vi "AlliGator Load HDF5 FLI Dataset Information.vi"(8 "Error In":errorcluster, 11 "File Path":path) -> (0 "error out":errorcluster, 1 "Data Description":string, 2 "Metadata":string, 3 "FLI Data File Information":T1, 4 "elapsed (relative) seconds":dbl)   [LabVIEW 2021, in "AlliGator HDF5.lvlib"]
doc: "Loads HDF5 FLI dataset information."
uses:
  AlliGator HDF5.lvlib
  AlliGator FLI Data File Information.ctl
  Phasor/Phasor Fluorescence Lifetime Parameters v3.ctl
  Files/AlliGator FLI Dataset Type.ctl
  AlliGator HDF5 FLI File Loading Information v0.6.ctl
  AlliGator HDF5 FLI File Loading Information v0.2.ctl
  Phasor/Fluorescence Lifetime Parameters.ctl
  SwissSPAD/SwissSPAD Live_Image ROI Information.ctl
  Source Image/AlliGator Image Binning Options.ctl
  Phasor/Phasor Fluorescence Lifetime Parameters v2.ctl
  <vilib>/addons/h5labview2/base/lib_path.vi
  <vilib>/addons/h5labview2/base/H5Equery.vi
  <vilib>/Utility/error.llb/Error Cluster From Error Code.vi
  AlliGator Load Single HDF5 Gate Image v 0.2b.vi
  AlliGator Load Single HDF5 Gate Image v 0.3b.vi
  AlliGator Load Single Gate Image from HDF5 v 0.6b.vi
  <vilib>/addons/h5labview2/base/hid_t.ctl
  <vilib>/addons/h5labview2/dataset/H5Dread.llb/H5Dread.xnode
  <vilib>/ErrorRing/Error Ring.xnode
  <vilib>/addons/h5labview2/file/H5F.lvlib
  <vilib>/addons/h5labview2/group/H5G.lvlib
  Time/Time.lvlib
  Phasor/Phasor.lvlib
  SwissSPAD/SwissSPAD Live.lvlib
  Source Image/AlliGator Source Image.lvlib
  Files/AlliGator Files.lvlib
  Variant/Variant.lvlib
panel:
  # "see the AlliGator License on the block diagram (Ctrl+E or Window:Show Block Diagram)"
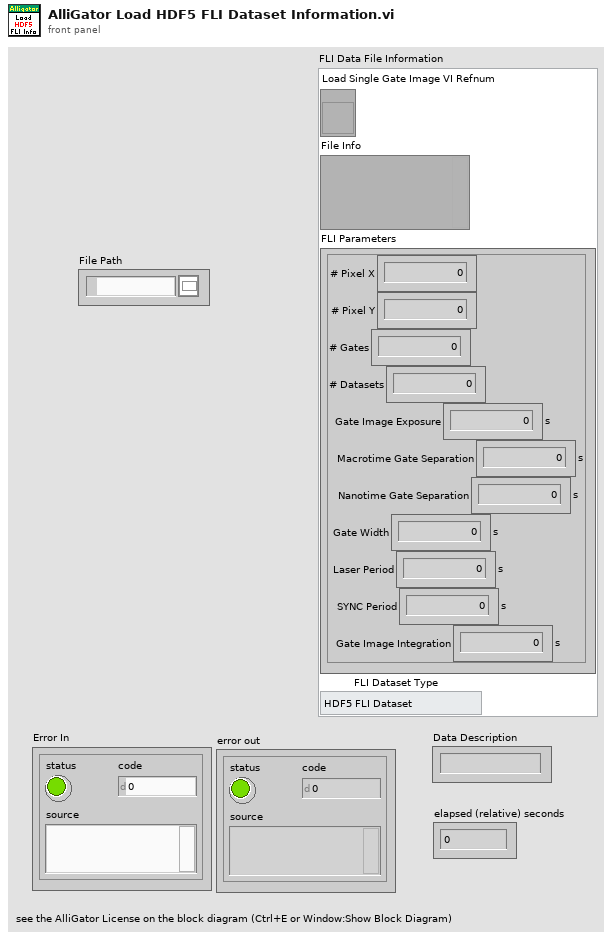
[diagram p1: front panel]
types:
  T1 = typedef "AlliGator HDF5.lvlib/AlliGator FLI Data File Information.ctl" = cluster{"Load Single Gate Image VI Refnum":refnum<vi>, "File Info":variant, "FLI Parameters":T2, "FLI Dataset Type":T3}
  T2 = typedef "Phasor.lvlib/Phasor Fluorescence Lifetime Parameters v3.ctl" = cluster{"# Pixel X":i32, "# Pixel Y":i32, "# Gates":i32, "# Datasets":i32, "Gate Image Exposure":dbl[unit], "Macrotime Gate Separation":dbl[unit], "Nanotime Gate Separation":dbl[unit], "Gate Width":dbl[unit], "Laser Period":dbl[unit], "SYNC Period":dbl[unit], "Gate Image Integration":dbl[unit]}
  T3 = typedef "AlliGator Files.lvlib/AlliGator FLI Dataset Type.ctl" = enum16{"HDF5 FLI Dataset", "Gate Image Folder", ".sdt FLI Dataset (Becker & Hickl)", ".ptu FLI Dataset (PicoQuant)", "SS1 FLI Dataset", "SS2 FLI Dataset", "I/m/phi Dataset", ".bin FLI Dataset (PicoQuant Binned)", ".bin FLI Dataset (Piccolo Binned)"}
  T4 = typedef "AlliGator HDF5.lvlib/AlliGator HDF5 FLI File Loading Information v0.6.ctl" = cluster{"HDF5 File Path":path, "Data Type":string, "# Datasets in Series":i32, "Dataset ID in Series":i32, "Channel Names":string[]}
  T5 = typedef "Phasor.lvlib/Fluorescence Lifetime Parameters.ctl" = cluster{"# Pixel X":i32, "# Pixel Y":i32, "# Gates":i32, "# Datasets":i32, "Exposure/Gate":dbl[unit], "Macrotime Gate Separation":dbl[unit], "Nanotime Gate Separation":dbl[unit], "Gate Duration":dbl[unit], "Laser Period":dbl[unit]}
  T6 = typedef "AlliGator HDF5.lvlib/AlliGator HDF5 FLI File Loading Information v0.2.ctl" = cluster{"HDF5 File Path":path}
  T7 = typedef "AlliGator Source Image.lvlib/AlliGator Image Binning Options.ctl" = cluster{"Use Image Binning":bool, "X Bin":i32, "Y Bin":i32}
  T8 = typedef "SwissSPAD Live.lvlib/SwissSPAD Live_Image ROI Information.ctl" = cluster{"Save ROI Only":bool, "Left":u16, "Top":u16, "Right":u16, "Bottom":u16, "Use Current ROI":bool}
  T9 = typedef "Phasor.lvlib/Phasor Fluorescence Lifetime Parameters v2.ctl" = cluster{"# Pixel X":i32, "# Pixel Y":i32, "# Gates":i32, "# Datasets":i32, "Exposure/Gate":dbl[unit], "Macrotime Gate Separation":dbl[unit], "Nanotime Gate Separation":dbl[unit], "Gate Duration":dbl[unit], "Laser Period":dbl[unit], "SYNC Period":dbl[unit]}
  T10 = typedef "hid_t.ctl" = i64
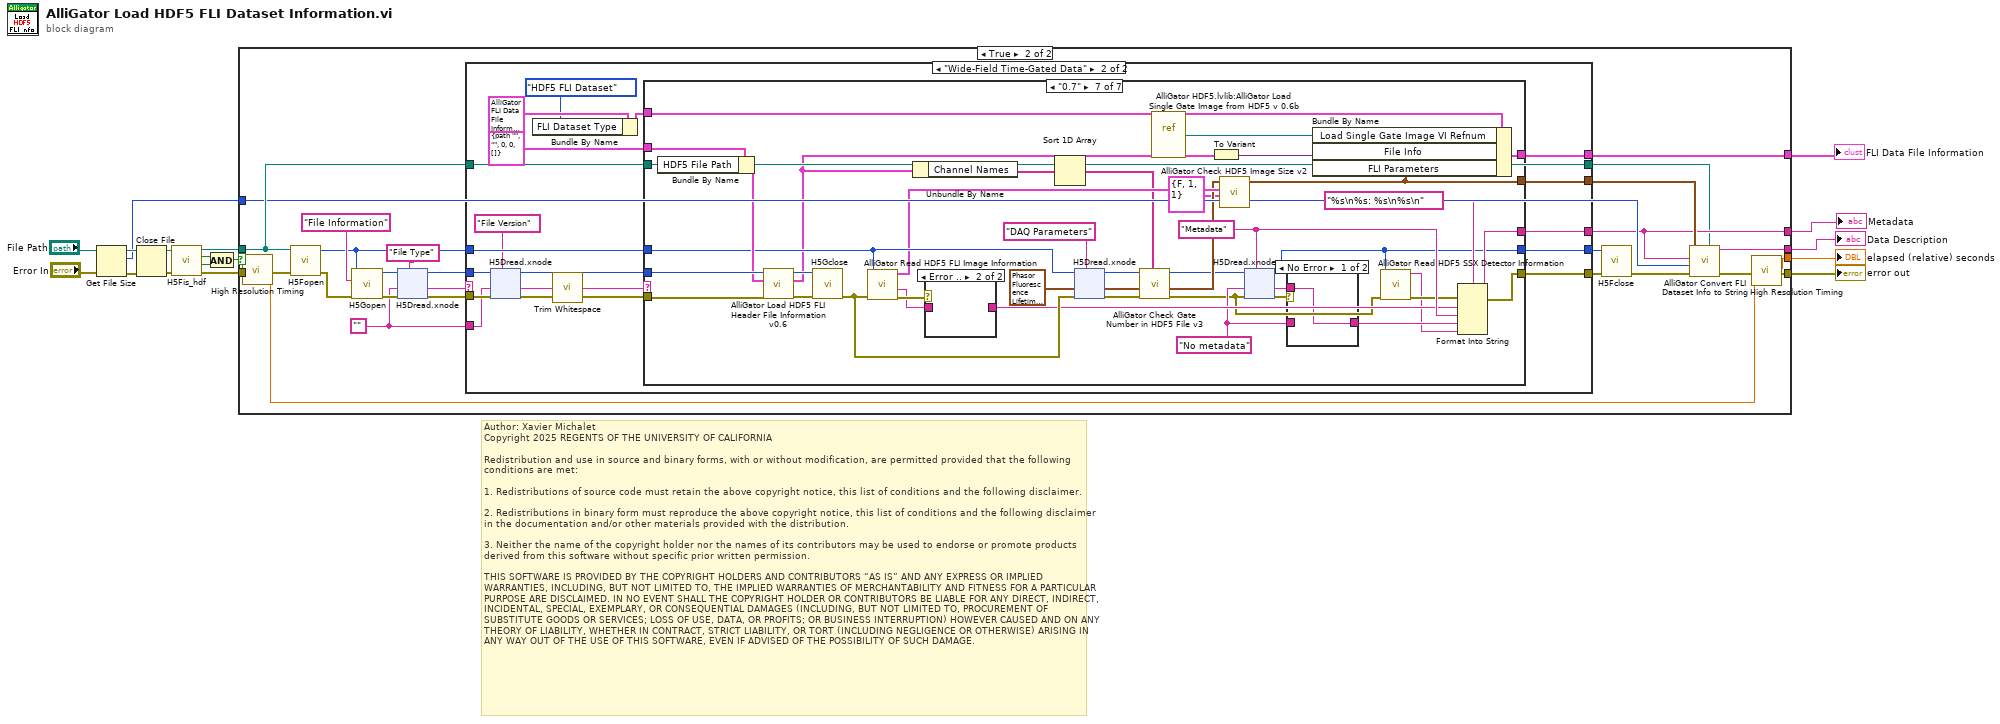
[diagram p0: block diagram]
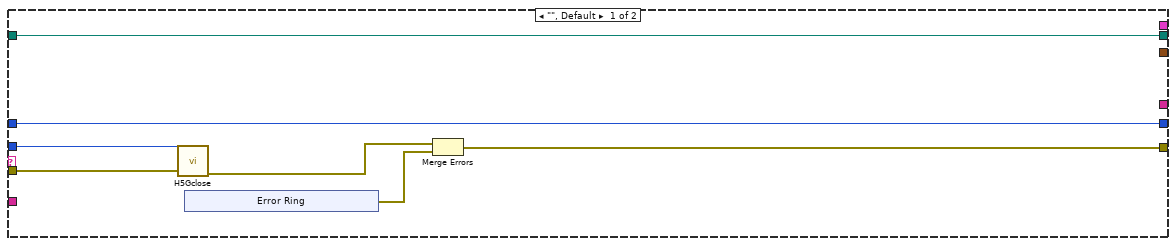
[diagram p3: hidden frame]
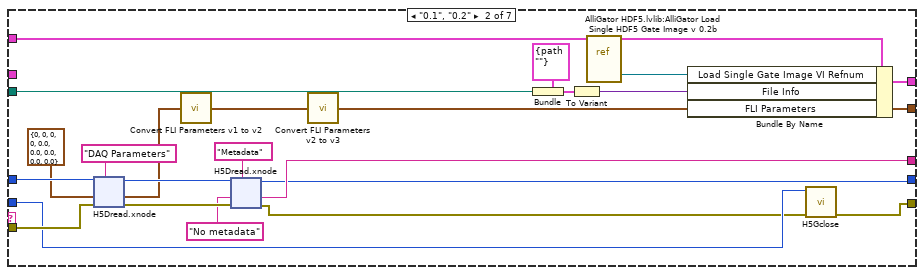
[diagram p5: hidden frame]
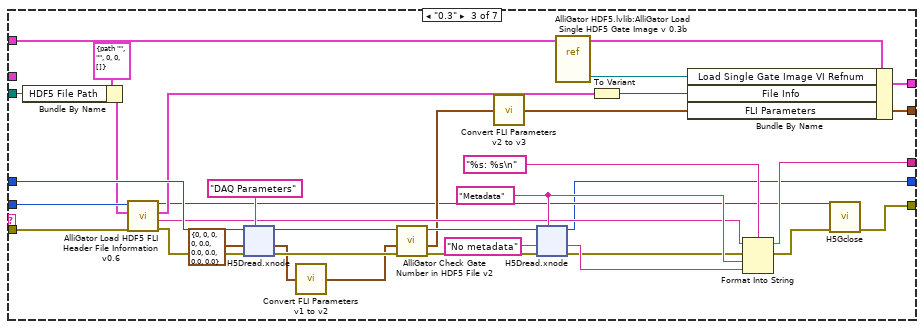
[diagram p6: hidden frame]
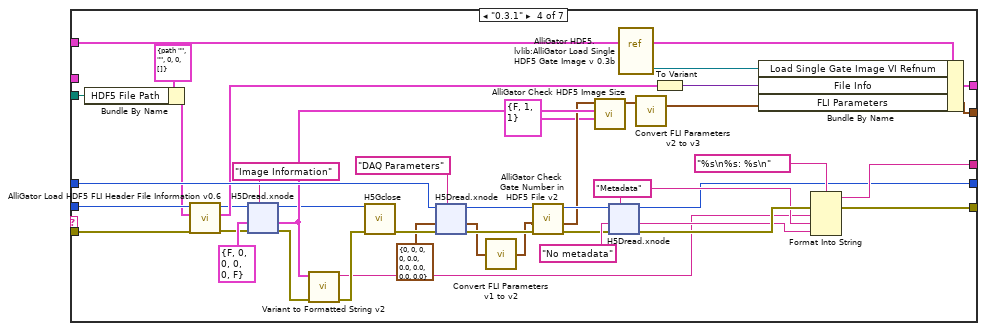
[diagram p7: hidden frame]
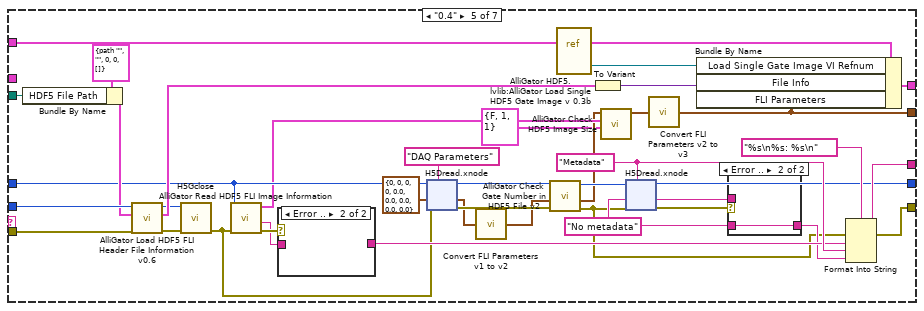
[diagram p8: hidden frame]
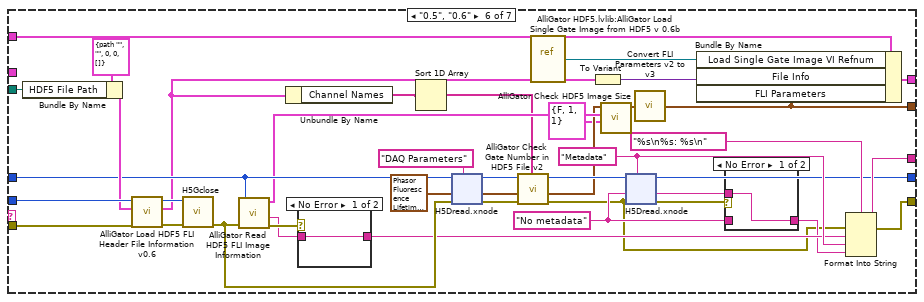
[diagram p11: hidden frame]
diagram:
  # "Author: Xavier Michalet\nCopyright 2025 REGENTS OF THE UNIVERSITY OF CALIFORNIA\n\nRedistribution and use in source and binary forms, with or without modification, are permitted provided that the following conditions are met:\n\n1. Redistributions of source code must retain the above copyright notice, this list of conditions and the following disclaimer.\n\n2. Redistributions in binary form must reproduce the above copyright notice, this list of conditions and the following disclaimer in the documentation and/or other materials provided with the distribution.\n\n3. Neither the name of the copyright holder nor the names of its contributors may be used to endorse or promote products derived from this software without specific prior written permission.\n\nTHIS SOFTWARE IS PROVIDED BY THE COPYRIGHT HOLDERS AND CONTRIBUTORS “AS IS” AND ANY EXPRESS OR IMPLIED WARRANTIES, INCLUDING, BUT NOT LIMITED TO, THE IMPLIED WARRANTIES OF MERCHANTABILITY AND FITNESS FOR A PARTICULAR PURPOSE ARE DISCLAIMED. IN NO EVENT SHALL THE COPYRIGHT HOLDER OR CONTRIBUTORS BE LIABLE FOR ANY DIRECT, INDIRECT, INCIDENTAL, SPECIAL, EXEMPLARY, OR CONSEQUENTIAL DAMAGES (INCLUDING, BUT NOT LIMITED TO, PROCUREMENT OF SUBSTITUTE GOODS OR SERVICES; LOSS OF USE, DATA, OR PROFITS; OR BUSINESS INTERRUPTION) HOWEVER CAUSED AND ON ANY THEORY OF LIABILITY, WHETHER IN CONTRACT, STRICT LIABILITY, OR TORT (INCLUDING NEGLIGENCE OR OTHERWISE) ARISING IN ANY WAY OUT OF THE USE OF THIS SOFTWARE, EVEN IF ADVISED OF THE POSSIBILITY OF SUCH DAMAGE."
  n1 = Get File Size(file="File Path", error in="Error In") -> (refnum out=w8:refnum<file>, size (in bytes)=w2:i64, 0:w9:errorcluster)
  n2 = Close File(refnum=w8, error in=w9) -> (path=w7:path, error out=w6:errorcluster)
  n3 = call <vilib>:"H5Fis_hdf.vi"("error in (no error)"=w6, "path in"=w7) -> ("error out"=w13:errorcluster, "valid?"=w16:bool, "exists?"=w17:bool, "path out"=w14:path)  [unwired: 6 in]
  n4 = And(x=w17, y=w16) -> (x .and. y?=w15:bool)
  n5 = case shown="True" w15 {
    tunnel: w14 -> [_ w27]
    tunnel: w13 -> [w18 w44]
    tunnel: [w18 w39] -> w12
    tunnel: [_ w37] -> w5
    tunnel: [_ w21] -> w4
    tunnel: [_ w26] -> w3
    tunnel: w2 -> [_ w23]
    tunnel: [_ w20] -> w1
    frame False {
    }
    frame True {
      w28 = ""
      n6 = call "High Resolution Timing.vi"("Error In"=w44) -> ("elapsed (relative) seconds"=w38:dbl, "Error Out"=w40:errorcluster)  [unwired: 16 in, 1 out]
      n7 = call <vilib>:"H5Fopen.vi"("error in (no error)"=w40, "path"=w27) -> ("error out"=w36:errorcluster, "ref out"=w31:T10)  [unwired: 8 in]
      n8 = call <vilib>:"H5Gopen.vi"("error in (no error)"=w36, "name"="File Information" ("dataset name (this)"), "ref in"=w31) -> ("error out"=w34:errorcluster, "group out"=w33:T10)  [unwired: 7 in]
      n9 = xnode "H5Dread.xnode"("dataset name (this)"="File Type", "error in (no error)"=w34, "default"=w28, "ref in"=w33) -> ("error out"=w30:errorcluster, "data"=w43:string, "ref out"=w29:T10)  [unwired: 2 in, 1 out]
      n10 = case shown="\"Wide-Field Time-Gated Data\"" w43 {
        tunnel: [w66 w89] -> w42
        tunnel: [w61 w75] -> w41
        tunnel: w31 -> [w66 w88]
        tunnel: w30 -> [w65 w86]
        tunnel: w28 -> [_ w85]
        tunnel: w29 -> [w64 w84]
        tunnel: [_ w82] -> w21
        tunnel: w27 -> [w62 w76]
        tunnel: [_ w80] -> w26
        tunnel: [_ w77] -> w22
        tunnel: [w62 w76] -> w19
        frame "", Default {
          n11 = call <vilib>:"H5Gclose.vi"("error in (no error)"=w65, "group in"=w64) -> ("error out"=w63:errorcluster)  [unwired: 9 in]
          n12 = xnode "Error Ring"() -> ("error out"=w60:errorcluster)
          n13 = Merge Errors(w63, w60) -> (w61:errorcluster)
        }
        frame "Wide-Field Time-Gated Data" {
          n14 = xnode "H5Dread.xnode"("dataset name (this)"="File Version", "error in (no error)"=w86, "default"=w85, "ref in"=w84) -> ("error out"=w79:errorcluster, "data"=w83:string, "ref out"=w78:T10)  [unwired: 2 in, 1 out]
          n15 = Bundle By Name(cluster=T1 {"Load Single Gate Image VI Refnum"=refnum, "File Info"=variant, "FLI Parameters"={"# Pixel X"=0, "# Pixel Y"=0, "# Gates"=0, "# Datasets"=0, "Gate Image Exposure"=0.0, "Macrotime Gate Separation"=0.0, "Nanotime Gate Separation"=0.0, "Gate Width"=0.0, "Laser Period"=0.0, "SYNC Period"=0.0, "Gate Image Integration"=0.0}, "FLI Dataset Type"=enum."HDF5 FLI Dataset"} ("FLI Data File Information"), "FLI Dataset Type"=AlliGator_FLI_Dataset_Type."HDF5 FLI Dataset") -> (w74:T1)
          n16 = call <vilib>:"Trim Whitespace.vi"("string"=w83) -> ("trimmed string"=w72:string)  [unwired: 1 in]
          n17 = case shown="\"0.7\"" w72 {
            tunnel: w88 -> [w106 w128 w192 w263 w326 w401 w478]
            tunnel: w79 -> [w105 w129 w184 w255 w340 w414 w488]
            tunnel: [w106 w108 w160 w241 w329 w404 w461] -> w89
            tunnel: [w105 w112 w166 w227 w337 w411 w485] -> w75
            tunnel: [_ w122 w181 w253 w338 w412 w486] -> w82
            tunnel: w74 -> [_ w121 w188 w259 w344 w417 w491]
            tunnel: w76 -> [_ w120 w182 w254 w339 w413 w487]
            tunnel: [_ w118 w186 w257 w342 w416 w490] -> w80
            tunnel: w78 -> [_ w113 w185 w256 w341 w415 w489]
            tunnel: [_ w109 w162 w223 w309 w383 w462] -> w77
            tunnel: T4 {"HDF5 File Path"=path "", "Data Type"="", "# Datasets in Series"=0, "Dataset ID in Series"=0, "Channel Names"=[]} ("output cluster") -> [_ _ _ _ _ _ w454]
            frame "", Default {
            }
            frame "0.1", "0.2" {
              n18 = xnode "H5Dread.xnode"("dataset name (this)"="DAQ Parameters", "error in (no error)"=w129, "default"=T5 {"# Pixel X"=0, "# Pixel Y"=0, "# Gates"=0, "# Datasets"=0, "Exposure/Gate"=0.0, "Macrotime Gate Separation"=0.0, "Nanotime Gate Separation"=0.0, "Gate Duration"=0.0, "Laser Period"=0.0} ("FLI Parameters"), "ref in"=w128) -> ("error out"=w126:errorcluster, "data"=w117:T5, "ref out"=w125:i64)  [unwired: 2 in, 1 out]
              n19 = call "Convert FLI Parameters v1 to v2.vi"("FLI Parameters"=w117) -> ("FLI Parameters v2"=w110:T9)  [unwired: 8 in]
              n20 = xnode "H5Dread.xnode"("dataset name (this)"="Metadata" ("dataset name"), "error in (no error)"=w126, "default"="No metadata" ("type name (default)"), "ref in"=w125) -> ("error out"=w107:errorcluster, "data"=w122:string, "ref out"=w108:T10)  [unwired: 2 in, 1 out]
              n21 = call "Convert FLI Parameters v2 to v3.vi"("FLI Parameters v2"=w110) -> ("FLI Parameters v3"=w109:T2)
              n22 = Bundle(cluster=T6 {"HDF5 File Path"=path ""} ("output cluster"), "HDF5 File Path"=w120) -> (w115:T6)
              n23 = To Variant(anything=w115) -> (Variant=w116:variant)
              n24 = vi-ref "AlliGator HDF5.lvlib:AlliGator Load Single HDF5 Gate Image v 0.2b.vi"() -> (w119:refnum<vi>)
              n25 = Bundle By Name(cluster=w121, "Load Single Gate Image VI Refnum"=w119, "File Info"=w116, "FLI Parameters"=w109) -> (w118:T1)
              n26 = call <vilib>:"H5Gclose.vi"("error in (no error)"=w107, "group in"=w113) -> ("error out"=w112:errorcluster)  [unwired: 9 in]
            }
            frame "0.3" {
              w180 = "Metadata" ("dataset name")
              n27 = Bundle By Name(cluster=T4 {"HDF5 File Path"=path "", "Data Type"="", "# Datasets in Series"=0, "Dataset ID in Series"=0, "Channel Names"=[]} ("output cluster"), "HDF5 File Path"=w182) -> (w173:T4)
              n28 = call "AlliGator Load HDF5 FLI Header File Information v0.6.vi"("error in (no error)"=w184, "HDF5 FLI File Loading Information"=w173, "ref in"=w185) -> ("error out"=w183:errorcluster, "File Information String"=w175:string, "HDF5 FLI File Loading Information out"=w172:T4, "ref out"=w167:T10)  [unwired: 5 in]
              n29 = xnode "H5Dread.xnode"("dataset name (this)"="DAQ Parameters", "error in (no error)"=w183, "default"=T5 {"# Pixel X"=0, "# Pixel Y"=0, "# Gates"=0, "# Datasets"=0, "Exposure/Gate"=0.0, "Macrotime Gate Separation"=0.0, "Nanotime Gate Separation"=0.0, "Gate Duration"=0.0, "Laser Period"=0.0} ("FLI Parameters"), "ref in"=w192) -> ("error out"=w190:errorcluster, "data"=w164:T5, "ref out"=w189:T10)  [unwired: 2 in, 1 out]
              n30 = call "Convert FLI Parameters v1 to v2.vi"("FLI Parameters"=w164) -> ("FLI Parameters v2"=w163:T9)  [unwired: 8 in]
              n31 = call "AlliGator Check Gate Number in HDF5 File v2.vi"("error in (no error)"=w190, "FLI Parameters"=w163, "ref in"=w189) -> ("error out"=w171:errorcluster, "FLI Parameters"=w169:T9, "ref"=w170:T10)  [unwired: 4 in, 2 out]
              n32 = call "Convert FLI Parameters v2 to v3.vi"("FLI Parameters v2"=w169) -> ("FLI Parameters v3"=w162:T2)
              n33 = xnode "H5Dread.xnode"("dataset name (this)"=w180, "error in (no error)"=w171, "default"="No metadata" ("type name (default)"), "ref in"=w170) -> ("error out"=w161:errorcluster, "data"=w178:string, "ref out"=w160:T10)  [unwired: 2 in, 1 out]
              n34 = vi-ref "AlliGator HDF5.lvlib:AlliGator Load Single HDF5 Gate Image v 0.3b.vi"() -> (w187:refnum<vi>)
              n35 = To Variant(anything=w172) -> (Variant=w177:variant)
              n36 = Bundle By Name(cluster=w188, "Load Single Gate Image VI Refnum"=w187, "File Info"=w177, "FLI Parameters"=w162) -> (w186:T1)
              n37 = Format Into String(format string="%s: %s\n", initial string=w175, error in=w161, w180, w178) -> (resulting string=w181:string, error out=w168:errorcluster)
              n38 = call <vilib>:"H5Gclose.vi"("error in (no error)"=w168, "group in"=w167) -> ("error out"=w166:errorcluster)  [unwired: 9 in]
            }
            frame "0.3.1" {
              w244 = "Metadata" ("dataset name")
              n39 = Bundle By Name(cluster=T4 {"HDF5 File Path"=path "", "Data Type"="", "# Datasets in Series"=0, "Dataset ID in Series"=0, "Channel Names"=[]} ("output cluster"), "HDF5 File Path"=w254) -> (w247:T4)
              n40 = call "AlliGator Load HDF5 FLI Header File Information v0.6.vi"("error in (no error)"=w255, "HDF5 FLI File Loading Information"=w247, "ref in"=w256) -> ("error out"=w236:errorcluster, "HDF5 FLI File Loading Information out"=w246:T4, "ref out"=w237:T10)  [unwired: 5 in, 1 out]
              n41 = xnode "H5Dread.xnode"("dataset name (this)"="Image Information" ("name"), "error in (no error)"=w236, "default"=T8 {"Save ROI Only"=FALSE, "Left"=0, "Top"=0, "Right"=0, "Bottom"=0, "Use Current ROI"=FALSE} ("Image Information"), "ref in"=w237) -> ("error out"=w238:errorcluster, "data"=w234:T8, "ref out"=w231:T10)  [unwired: 2 in, 1 out]
              n42 = call "Variant to Formatted String v2.vi"("error in (no error)"=w238, "Anything"=w234) -> ("error out"=w230:errorcluster, "String"=w228:string)  [unwired: 8 in]
              n43 = call <vilib>:"H5Gclose.vi"("error in (no error)"=w230, "group in"=w231) -> ("error out"=w229:errorcluster)  [unwired: 9 in]
              n44 = xnode "H5Dread.xnode"("dataset name (this)"="DAQ Parameters", "error in (no error)"=w229, "default"=T5 {"# Pixel X"=0, "# Pixel Y"=0, "# Gates"=0, "# Datasets"=0, "Exposure/Gate"=0.0, "Macrotime Gate Separation"=0.0, "Nanotime Gate Separation"=0.0, "Gate Duration"=0.0, "Laser Period"=0.0} ("FLI Parameters"), "ref in"=w263) -> ("error out"=w261:errorcluster, "data"=w225:T5, "ref out"=w260:T10)  [unwired: 2 in, 1 out]
              n45 = call "Convert FLI Parameters v1 to v2.vi"("FLI Parameters"=w225) -> ("FLI Parameters v2"=w224:T9)  [unwired: 8 in]
              n46 = call "AlliGator Check Gate Number in HDF5 File v2.vi"("error in (no error)"=w261, "FLI Parameters"=w224, "ref in"=w260) -> ("error out"=w243:errorcluster, "FLI Parameters"=w233:T9, "ref"=w242:T10)  [unwired: 4 in, 2 out]
              n47 = call "AlliGator Check HDF5 Image Size.vi"("Image Binning Options"=T7 {"Use Image Binning"=FALSE, "X Bin"=1, "Y Bin"=1}, "Image ROI Information"=w234, "FLI Parameters in"=w233) -> ("FLI Parameters out"=w235:T9)  [unwired: 8 in]
              n48 = xnode "H5Dread.xnode"("dataset name (this)"=w244, "error in (no error)"=w243, "default"="No metadata" ("type name (default)"), "ref in"=w242) -> ("error out"=w252:errorcluster, "data"=w245:string, "ref out"=w241:T10)  [unwired: 2 in, 1 out]
              n49 = vi-ref "AlliGator HDF5.lvlib:AlliGator Load Single HDF5 Gate Image v 0.3b.vi"() -> (w258:refnum<vi>)
              n50 = call "Convert FLI Parameters v2 to v3.vi"("FLI Parameters v2"=w235) -> ("FLI Parameters v3"=w223:T2)
              n51 = To Variant(anything=w246) -> (Variant=w250:variant)
              n52 = Bundle By Name(cluster=w259, "Load Single Gate Image VI Refnum"=w258, "File Info"=w250, "FLI Parameters"=w223) -> (w257:T1)
              n53 = Format Into String(format string="%s\n%s: %s\n", error in=w252, w228, w244, w245) -> (resulting string=w253:string, error out=w227:errorcluster)  [unwired: 1 in]
            }
            frame "0.4" {
              w312 = "No metadata" ("type name (default)")
              w331 = "Metadata" ("dataset name")
              n54 = Bundle By Name(cluster=T4 {"HDF5 File Path"=path "", "Data Type"="", "# Datasets in Series"=0, "Dataset ID in Series"=0, "Channel Names"=[]} ("output cluster"), "HDF5 File Path"=w339) -> (w333:T4)
              n55 = call "AlliGator Load HDF5 FLI Header File Information v0.6.vi"("error in (no error)"=w340, "HDF5 FLI File Loading Information"=w333, "ref in"=w341) -> ("error out"=w327:errorcluster, "HDF5 FLI File Loading Information out"=w332:T4, "ref out"=w328:T10)  [unwired: 5 in, 1 out]
              n56 = call <vilib>:"H5Gclose.vi"("error in (no error)"=w327, "group in"=w328) -> ("error out"=w315:errorcluster)  [unwired: 9 in]
              n57 = call "AlliGator Read HDF5 FLI Image Information.vi"("error in (no error)"=w315, "ref in"=w326) -> ("error out"=w318:errorcluster, "Image Information"=w317:string, "Image ROI Information"=w325:T8)  [unwired: 6 in, 1 out]
              n58 = case shown="Error .." w318 {
                tunnel: [w380 _] -> w316
                tunnel: w317 -> [w380 _]
                frame No Error {
                }
                frame Error {
                }
              }
              n59 = xnode "H5Dread.xnode"("dataset name (this)"="DAQ Parameters", "error in (no error)"=w315, "default"=T5 {"# Pixel X"=0, "# Pixel Y"=0, "# Gates"=0, "# Datasets"=0, "Exposure/Gate"=0.0, "Macrotime Gate Separation"=0.0, "Nanotime Gate Separation"=0.0, "Gate Duration"=0.0, "Laser Period"=0.0} ("FLI Parameters"), "ref in"=w326) -> ("error out"=w346:errorcluster, "data"=w320:T5, "ref out"=w345:T10)  [unwired: 2 in, 1 out]
              n60 = call "Convert FLI Parameters v1 to v2.vi"("FLI Parameters"=w320) -> ("FLI Parameters v2"=w319:T9)  [unwired: 8 in]
              n61 = call "AlliGator Check Gate Number in HDF5 File v2.vi"("error in (no error)"=w346, "FLI Parameters"=w319, "ref in"=w345) -> ("error out"=w310:errorcluster, "FLI Parameters"=w324:T9, "ref"=w330:T10)  [unwired: 4 in, 2 out]
              n62 = vi-ref "AlliGator HDF5.lvlib:AlliGator Load Single HDF5 Gate Image v 0.3b.vi"() -> (w343:refnum<vi>)
              n63 = To Variant(anything=w332) -> (Variant=w336:variant)
              n64 = call "AlliGator Check HDF5 Image Size.vi"("Image Binning Options"=T7 {"Use Image Binning"=FALSE, "X Bin"=1, "Y Bin"=1}, "Image ROI Information"=w325, "FLI Parameters in"=w324) -> ("FLI Parameters out"=w323:T9)  [unwired: 8 in]
              n65 = xnode "H5Dread.xnode"("dataset name (this)"=w331, "error in (no error)"=w310, "default"=w312, "ref in"=w330) -> ("error out"=w313:errorcluster, "data"=w314:string, "ref out"=w329:T10)  [unwired: 2 in, 1 out]
              n66 = call "Convert FLI Parameters v2 to v3.vi"("FLI Parameters v2"=w323) -> ("FLI Parameters v3"=w309:T2)
              n67 = Bundle By Name(cluster=w344, "Load Single Gate Image VI Refnum"=w343, "File Info"=w336, "FLI Parameters"=w309) -> (w342:T1)
              n68 = case shown="Error .." w313 {
                tunnel: [w378 w379] -> w311
                tunnel: w312 -> [_ w379]
                tunnel: w314 -> [w378 _]
                frame No Error {
                }
                frame Error {
                }
              }
              n69 = Format Into String(format string="%s\n%s: %s\n", error in=w310, w316, w331, w311) -> (resulting string=w338:string, error out=w337:errorcluster)  [unwired: 1 in]
            }
            frame "0.5", "0.6" {
              w389 = "No metadata" ("type name (default)")
              w406 = "Metadata" ("dataset name")
              n70 = Bundle By Name(cluster=T4 {"HDF5 File Path"=path "", "Data Type"="", "# Datasets in Series"=0, "Dataset ID in Series"=0, "Channel Names"=[]} ("output cluster"), "HDF5 File Path"=w413) -> (w407:T4)
              n71 = call "AlliGator Load HDF5 FLI Header File Information v0.6.vi"("error in (no error)"=w414, "HDF5 FLI File Loading Information"=w407, "ref in"=w415) -> ("error out"=w402:errorcluster, "HDF5 FLI File Loading Information out"=w384:T4, "ref out"=w403:T10)  [unwired: 5 in, 1 out]
              n72 = call <vilib>:"H5Gclose.vi"("error in (no error)"=w402, "group in"=w403) -> ("error out"=w393:errorcluster)  [unwired: 9 in]
              n73 = call "AlliGator Read HDF5 FLI Image Information.vi"("error in (no error)"=w393, "ref in"=w401) -> ("error out"=w394:errorcluster, "Image Information"=w392:string, "Image ROI Information"=w400:T8)  [unwired: 6 in, 1 out]
              n74 = Unbundle By Name(w384) -> ("Channel Names"=w382:string[])
              n75 = case shown="No Error" w394 {
                tunnel: [w453 _] -> w391
                tunnel: w392 -> [w453 _]
                frame No Error {
                }
                frame Error {
                }
              }
              n76 = Sort 1D Array(array=w382) -> (sorted array=w381:string[])
              n77 = xnode "H5Dread.xnode"("dataset name (this)"="DAQ Parameters", "error in (no error)"=w393, "default"=T9 {"# Pixel X"=0, "# Pixel Y"=0, "# Gates"=0, "# Datasets"=0, "Exposure/Gate"=0.0, "Macrotime Gate Separation"=0.0, "Nanotime Gate Separation"=0.0, "Gate Duration"=0.0, "Laser Period"=0.0, "SYNC Period"=0.0} ("Swiss SPAD File Information"), "ref in"=w401) -> ("error out"=w419:errorcluster, "data"=w395:T9, "ref out"=w418:i64)  [unwired: 2 in, 1 out]
              n78 = call "AlliGator Check Gate Number in HDF5 File v2.vi"("Gate Names"=w381, "error in (no error)"=w419, "FLI Parameters"=w395, "ref in"=w418) -> ("error out"=w386:errorcluster, "FLI Parameters"=w399:T9, "ref"=w405:T10)  [unwired: 3 in, 2 out]
              n79 = vi-ref "AlliGator HDF5.lvlib:AlliGator Load Single Gate Image from HDF5 v 0.6b.vi"() -> (w385:refnum<vi>)
              n80 = To Variant(anything=w384) -> (Variant=w410:variant)
              n81 = call "AlliGator Check HDF5 Image Size.vi"("Image Binning Options"=T7 {"Use Image Binning"=FALSE, "X Bin"=1, "Y Bin"=1}, "Image ROI Information"=w400, "FLI Parameters in"=w399) -> ("FLI Parameters out"=w398:T9)  [unwired: 8 in]
              n82 = xnode "H5Dread.xnode"("dataset name (this)"=w406, "error in (no error)"=w386, "default"=w389, "ref in"=w405) -> ("error out"=w390:errorcluster, "data"=w387:string, "ref out"=w404:T10)  [unwired: 2 in, 1 out]
              n83 = call "Convert FLI Parameters v2 to v3.vi"("FLI Parameters v2"=w398) -> ("FLI Parameters v3"=w383:T2)
              n84 = Bundle By Name(cluster=w417, "Load Single Gate Image VI Refnum"=w385, "File Info"=w410, "FLI Parameters"=w383) -> (w416:T1)
              n85 = case shown="No Error" w390 {
                tunnel: [w451 w452] -> w388
                tunnel: w389 -> [_ w452]
                tunnel: w387 -> [w451 _]
                frame No Error {
                }
                frame Error {
                }
              }
              n86 = Format Into String(format string="%s\n%s: %s\n", error in=w386, w391, w406, w388) -> (resulting string=w412:string, error out=w411:errorcluster)  [unwired: 1 in]
            }
            frame "0.7" {
              w467 = "No metadata" ("type name (default)")
              w481 = "Metadata" ("dataset name")
              n87 = Bundle By Name(cluster=w454, "HDF5 File Path"=w487) -> (w482:T4)
              n88 = call "AlliGator Load HDF5 FLI Header File Information v0.6.vi"("error in (no error)"=w488, "HDF5 FLI File Loading Information"=w482, "ref in"=w489) -> ("error out"=w479:errorcluster, "HDF5 FLI File Loading Information out"=w463:T4, "ref out"=w480:T10)  [unwired: 5 in, 1 out]
              n89 = call <vilib>:"H5Gclose.vi"("error in (no error)"=w479, "group in"=w480) -> ("error out"=w471:errorcluster)  [unwired: 9 in]
              n90 = call "AlliGator Read HDF5 FLI Image Information.vi"("error in (no error)"=w471, "ref in"=w478) -> ("error out"=w472:errorcluster, "Image Information"=w470:string, "Image ROI Information"=w477:T8)  [unwired: 6 in, 1 out]
              n91 = Unbundle By Name(w463) -> ("Channel Names"=w456:string[])
              n92 = case shown="Error .." w472 {
                tunnel: [w527 _] -> w469
                tunnel: w470 -> [w527 _]
                frame No Error {
                }
                frame Error {
                }
              }
              n93 = Sort 1D Array(array=w456) -> (sorted array=w455:string[])
              n94 = xnode "H5Dread.xnode"("dataset name (this)"="DAQ Parameters", "error in (no error)"=w471, "default"=T2 {"# Pixel X"=0, "# Pixel Y"=0, "# Gates"=0, "# Datasets"=0, "Gate Image Exposure"=0.0, "Macrotime Gate Separation"=0.0, "Nanotime Gate Separation"=0.0, "Gate Width"=0.0, "Laser Period"=0.0, "SYNC Period"=0.0, "Gate Image Integration"=0.0} ("Swiss SPAD File Information"), "ref in"=w478) -> ("error out"=w493:errorcluster, "data"=w473:T2, "ref out"=w492:T10)  [unwired: 2 in, 1 out]
              n95 = call "AlliGator Check Gate Number in HDF5 File v3.vi"("Gate Names"=w455, "error in (no error)"=w493, "FLI Parameters"=w473, "ref in"=w492) -> ("error out"=w460:errorcluster, "FLI Parameters"=w476:T2, "ref"=w457:T10)  [unwired: 3 in, 2 out]
              n96 = vi-ref "AlliGator HDF5.lvlib:AlliGator Load Single Gate Image from HDF5 v 0.6b.vi"() -> (w464:refnum<vi>)
              n97 = To Variant(anything=w463) -> (Variant=w484:variant)
              n98 = call "AlliGator Check HDF5 Image Size v2.vi"("Image Binning Options"=T7 {"Use Image Binning"=FALSE, "X Bin"=1, "Y Bin"=1}, "Image ROI Information"=w477, "FLI Parameters in"=w476) -> ("FLI Parameters out"=w462:T2)  [unwired: 8 in]
              n99 = xnode "H5Dread.xnode"("dataset name (this)"=w481, "error in (no error)"=w460, "default"=w467, "ref in"=w457) -> ("error out"=w468:errorcluster, "data"=w465:string, "ref out"=w461:T10)  [unwired: 2 in, 1 out]
              n100 = case shown="No Error" w468 {
                tunnel: [w525 w526] -> w466
                tunnel: w467 -> [_ w526]
                tunnel: w465 -> [w525 _]
                frame No Error {
                }
                frame Error {
                }
              }
              n101 = Bundle By Name(cluster=w491, "Load Single Gate Image VI Refnum"=w464, "File Info"=w484, "FLI Parameters"=w462) -> (w490:T1)
              n102 = call "AlliGator Read HDF5 SSX Detector Information.vi"("error in (no error)"=w460, "ref in"=w461) -> ("error out"=w459:errorcluster, "SwissSPAD Detector Information"=w458:string)  [unwired: 8 in]
              n103 = Format Into String(format string="%s\n%s: %s\n%s\n", error in=w459, w469, w481, w466, w458) -> (resulting string=w486:string, error out=w485:errorcluster)  [unwired: 1 in]
            }
          }
        }
      }
      n104 = call <vilib>:"H5Fclose.vi"("error in (no error)"=w41, "ref"=w42) -> ("error out"=w25:errorcluster)  [unwired: 9 in]
      n105 = call "AlliGator Convert FLI Dataset Info to String.vi"("File Path"=w19, "error in (no error)"=w25, "size"=w23, "Metadata"=w21, "FLI Parameters"=w22) -> ("Error Out"=w24:errorcluster, "Data Description"=w20:string)  [unwired: 5 in]
      n106 = call "High Resolution Timing.vi"("relative seconds (NaN)"=w38, "Error In"=w24) -> ("elapsed (relative) seconds"=w37:dbl, "Error Out"=w39:errorcluster)  [unwired: 15 in, 1 out]
    }
  }
  "error out" <- w12
  "elapsed (relative) seconds" <- w5
  "Metadata" <- w4
  "FLI Data File Information" <- w3
  "Data Description" <- w1
